vi "MT Measure CPM Quadrature Impairments.vi"(0 "recovered complex waveform":T5={"t0"=0.0, "dt"=1.0, "Y"=[]} {"Y" format="%.3f"; "dt" format="%^.2e"; "t0" format="%.4f"}, 1 "samples per symbol (16)":i32=16, 5 "detected complex waveform":cluster{"t0":dbl, "dt":dbl, "Y":cdb[]} {"Y" format="%.3f"; "dt" format="%^.2e"; "t0" format="%.4f"}, 7 "impairment measurement window":T3={"start index (symbols)"=0, "width (symbols) (-1: all)"=-1}, 11 "error in (no error)":errorcluster, 12 "impairment definition":enum16{"Vertical Shear", "Axis Shear"}(ring)) -> (2 "magnitude error":T1 {"individual symbol measurements (%)" format="%.2f"; "peak measurement (%)" format="%.2f"; "RMS measurement (%)" format="%.2f"}, 3 "DC offset measurements":T4 {"origin offset (dB)" format="%.2f"; "Q (%)" format="%.2f"; "I (%)" format="%.2f"}, 4 "IQ gain imbalance (dB)":dbl format="%.2f", 6 "phase error":T2 {"individual symbol measurements (deg)" format="%.2f"; "peak measurement (deg)" format="%.2f"; "RMS measurement (deg)" format="%.2f"}, 8 "EVM":T1 {"individual symbol measurements (%)" format="%.2f"; "peak measurement (%)" format="%.2f"; "RMS measurement (%)" format="%.2f"}, 10 "modulation error ratio (dB)":dbl format="%.2f", 14 "quadrature skew (deg)":dbl format="%.2f", 15 "error out":errorcluster)   [LabVIEW 2020, in "niDMT.lvlib"]
doc: "Measures and reports quadrature impairments over a single user-specified window. This VI must be called once for each measurement window. This polymorphic instance calculates continuous phase modulation (CPM) quadrature impairments on a point-by-point basis on the oversampled waveform."
uses:
  <vilib>/addons/Modulation/niDMT.lvlib
  <vilib>/addons/Modulation/Analog/controls/Complex Data Waveform.ctl
  <vilib>/addons/Modulation/niAMT.lvlib
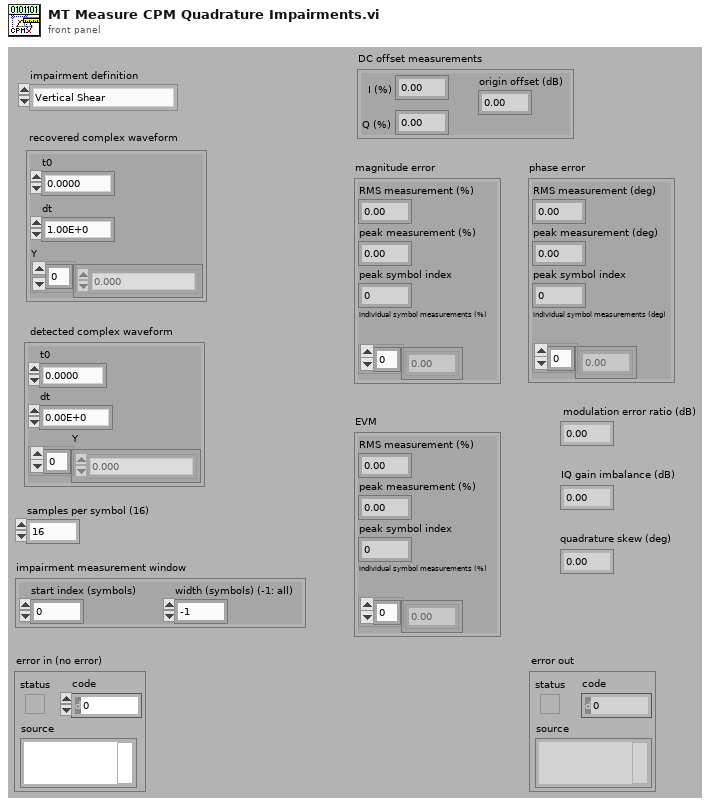
[diagram p1: front panel]
types:
  T1 = cluster{"RMS measurement (%)":dbl, "peak measurement (%)":dbl, "peak symbol index":i32, "individual symbol measurements (%)":dbl[]}
  T2 = cluster{"RMS measurement (deg)":dbl, "peak measurement (deg)":dbl, "peak symbol index":i32, "individual symbol measurements (deg)":dbl[]}
  T3 = cluster{"start index (symbols)":i32, "width (symbols) (-1: all)":i32}
  T4 = cluster{"I (%)":dbl, "Q (%)":dbl, "origin offset (dB)":dbl}
  T5 = typedef "niAMT.lvlib/Complex Data Waveform.ctl" = cluster{"t0":dbl, "dt":dbl, "Y":cdb[]}
  T6 = enum16{"FSK", "PSK", "QAM", "MSK", "PAM", "ASK", "CPM"}
  T7 = cluster{"I, %":dbl, "Q, %":dbl, "Origin Offset, dB":dbl}
  T8 = cluster{"RMS Measurement, deg":dbl, "Peak Measurement, deg":dbl, "Peak Symbol Index":i32, "Individual Symbol Measurements, deg":dbl[]}
  T9 = cluster{"RMS Measurement, %":dbl, "Peak Measurement, %":dbl, "Peak Symbol Index":i32, "Individual Symbol Measurements, %":dbl[]}
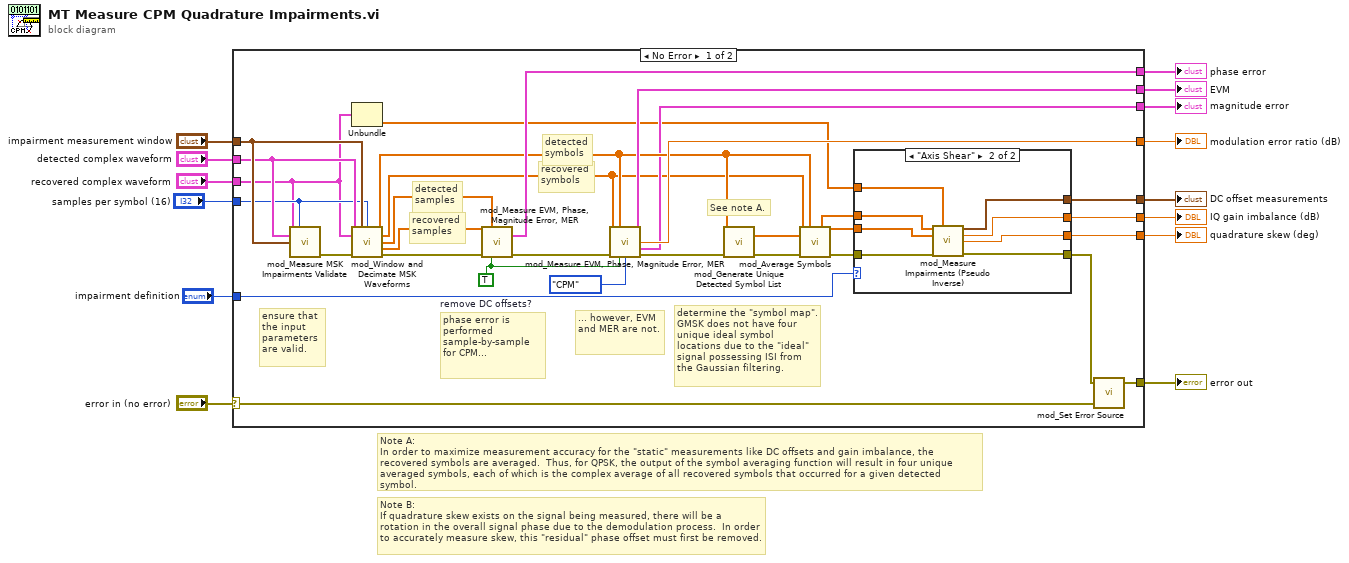
[diagram p0: block diagram]
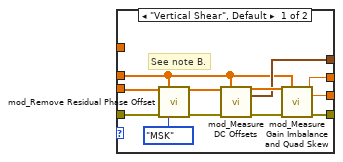
[diagram p2: hidden frame]
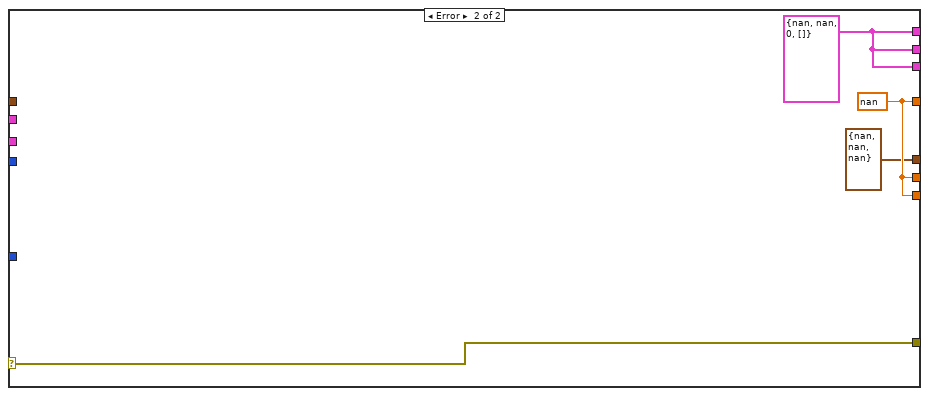
[diagram p3: hidden frame]
diagram:
  # "Note A:\nIn order to maximize measurement accuracy for the \"static\" measurements like DC offsets and gain imbalance, the recovered symbols are averaged.  Thus, for QPSK, the output of the symbol averaging function will result in four unique averaged symbols, each of which is the complex average of all recovered symbols that occurred for a given detected symbol."
  # "Note B:\nIf quadrature skew exists on the signal being measured, there will be a rotation in the overall signal phase due to the demodulation process.  In order to accurately measure skew, this \"residual\" phase offset must first be removed."
  n1 = case shown="No Error" "error in (no error)" {
    selector: "error in (no error)" -> [w43 w69]
    tunnel: "recovered complex waveform" -> [w17 _]
    tunnel: [w44 T7 {"I, %"=nan, "Q, %"=nan, "Origin Offset, dB"=nan} ("DC Offset Measurements")] -> w9
    tunnel: [w45 w68] -> w7
    tunnel: [w35 w68] -> w8
    tunnel: [w22 w67] -> w6
    tunnel: [w42 w69] -> w13
    tunnel: "detected complex waveform" -> [w31 _]
    tunnel: "impairment measurement window" -> [w32 _]
    tunnel: [w34 w67] -> w3
    tunnel: [w41 w67] -> w5
    tunnel: "samples per symbol (16)" -> [w30 _]
    tunnel: [w20 w68] -> w2
    tunnel: "impairment definition" -> [w19 _]
    frame No Error {
      w21 = TRUE  # remove DC offsets?
      # "See note A."
      # "ensure that the input parameters are valid."
      # "detected\nsamples"
      # "recovered\nsamples"
      # "recovered\nsymbols"
      # "detected\nsymbols"
      # "... however, EVM and MER are not."
      # "phase error is performed sample-by-sample for CPM..."
      # "determine the \"symbol map\".  GMSK does not have four unique ideal symbol locations due to the \"ideal\" signal possessing ISI from the Gaussian filtering."
      n2 = call <vilib>:"mod_Measure MSK Impairments Validate.vi"("Recovered Sample Sequence"=w17, "Samples Per Symbol (16)"=w30, "Detected Sample Sequence"=w31, "Impairment Measurement Window"=w32) -> ("error out"=w33:errorcluster)  [unwired: 11 out]
      n3 = Unbundle(w17) -> ("Y"=w16:cdb[])  [unwired: 2 out]
      n4 = call <vilib>:"mod_Window and Decimate MSK Waveforms.vi"("Detected Complex Waveform"=w31, "Impairment Measurement Window"=w32, "Samples Per Symbol (16)"=w30, "Recovered Complex Waveform"=w17, "error in (no error)"=w33) -> ("Windowed Detected Symbols"=w26:cdb[], "Windowed Recovered Symbols"=w15:cdb[], "Windowed Detected Samples"=w28:cdb[], "Windowed Recovered Samples"=w27:cdb[], "error out"=w29:errorcluster)  [unwired: 1 in, 5 out]
      n5 = call <vilib>:"mod_Measure EVM, Phase, Magnitude Error, MER.vi"("Recovered Signal"=w27, "Detected Signal"=w28, "error in (no error)"=w29, "remove DC offsets? (T)"=w21) -> ("Phase Error"=w45:T8, "error out"=w24:errorcluster)  [unwired: 2 in, 8 out]
      n6 = call <vilib>:"mod_Measure EVM, Phase, Magnitude Error, MER.vi"("Recovered Signal"=w15, "Detected Signal"=w26, "error in (no error)"=w24, "remove DC offsets? (T)"=w21, "Modulation Type"=T6."CPM") -> ("EVM"=w35:T9, "Modulation Error Ratio, dB"=w34:dbl, "magnitude error"=w20:T9, "error out"=w25:errorcluster)  [unwired: 1 in, 6 out]
      n7 = call <vilib>:"mod_Generate Unique Detected Symbol List.vi"("Detected Symbols"=w26, "error in (no error)"=w25) -> ("Unique Detected Symbols"=w36:cdb[], "error out"=w37:errorcluster)  [unwired: 12 out]
      n8 = call <vilib>:"mod_Average Symbols.vi"("Recovered Symbols"=w15, "Detected Symbols"=w26, "Symbol Map"=w36, "error in (no error)"=w37) -> ("Grouped Detected Symbols"=w38:cdb[], "Averaged Symbols"=w39:cdb[], "error out"=w40:errorcluster)  [unwired: 9 out]
      n9 = case shown="\"Axis Shear\"" w19 {
        tunnel: [w55 w62] -> w44
        tunnel: [w54 w60] -> w41
        tunnel: w40 -> [w53 w63]
        tunnel: w39 -> [w51 w64]
        tunnel: w38 -> [w50 w65]
        tunnel: [w48 w59] -> w23
        tunnel: [w47 w61] -> w22
        tunnel: w16 -> [_ w58]
        frame "Vertical Shear", Default {
          # "See note B."
          n10 = call <vilib>:"mod_Remove Residual Phase Offset.vi"("Averaged Symbols In"=w51, "Grouped Detected Symbols"=w50, "error in (no error)"=w53, "Modulation Type"=T6."MSK") -> ("Averaged Symbols Out"=w49:cdb[], "error out"=w52:errorcluster)  [unwired: 10 out]
          n11 = call <vilib>:"mod_Measure DC Offsets.vi"("Averaged Symbols"=w49, "Grouped Detected Symbols"=w50, "error in (no error)"=w52) -> ("Corrected Symbols"=w56:cdb[], "DC Offset Measurements"=w55:T7, "error out"=w57:errorcluster)  [unwired: 1 in, 9 out]
          n12 = call <vilib>:"mod_Measure Gain Imbalance and Quad Skew.vi"("Corrected Symbols"=w56, "Grouped Detected Symbols"=w50, "error in (no error)"=w57) -> ("IQ Gain Imbalance, dB"=w47:dbl, "Quadrature Skew, deg"=w54:dbl, "error out"=w48:errorcluster)  [unwired: 1 in, 9 out]
        }
        frame "Axis Shear" {
          n13 = call <vilib>:"mod_Measure Impairments (Pseudo Inverse).vi"("Grouped detected symbols"=w65, "Recovered Complex Waveform"=w58, "Averaged symbols"=w64, "error in (no error)"=w63) -> ("DC Offset Measurements"=w62:T7, "IQ gain imbalance (dB)"=w61:dbl, "quadrature skew (deg)"=w60:dbl, "error out"=w59:errorcluster)  [unwired: 8 out]
        }
      }
      n14 = call <vilib>:"mod_Set Error Source.vi"("initial error in (no error)"=w43, "final error in (no error)"=w23) -> ("error out"=w42:errorcluster)  [unwired: 3 out]
    }
    frame Error {
      w67 = nan ("Modulation Error Ratio, dB")
      w68 = T8 {"RMS Measurement, deg"=nan, "Peak Measurement, deg"=nan, "Peak Symbol Index"=0, "Individual Symbol Measurements, deg"=[]} ("Phase Error")
    }
  }
  "error out" <- w13
  "IQ gain imbalance (dB)" <- w6
  "quadrature skew (deg)" <- w5
  "modulation error ratio (dB)" <- w3
  "DC offset measurements" <- w9
  "EVM" <- w8
  "phase error" <- w7
  "magnitude error" <- w2
